vi "Inverter-DCread vi.vi"(0 "Numeric Control 6":dbl, 1 "Numeric Control 5":dbl, 2 "Numeric Control 4":dbl, 3 "Numeric Control 16":dbl, 4 "Numeric Control 15":dbl, 6 "Numeric Control 17":u32, 7 "Numeric Control 14":dbl, 8 "register values":u16[](array[numeric]), 9 "Numeric Control 13":dbl, 11 "Numeric Control 12":dbl) -> (10 "Numeric Control 3":dbl, 12 "Numeric Control 2":dbl, 13 "Numeric Control 7":dbl, 14 "Numeric Control":dbl, 15 "Numeric Control 10":dbl, 16 "Numeric Control 11":dbl, 17 "Numeric Control 9":dbl, 18 "Numeric Control 8":dbl)   [LabVIEW 2016]
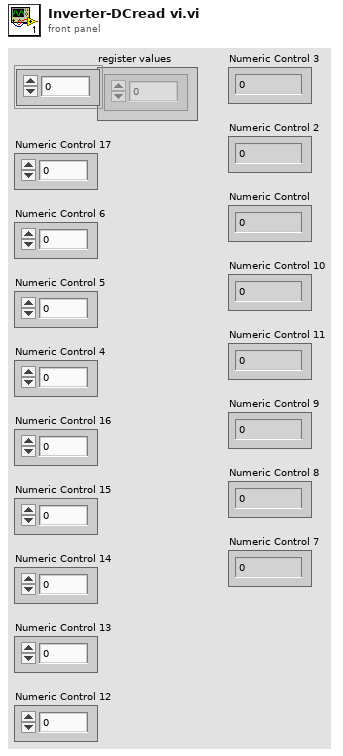
[diagram p1: front panel]
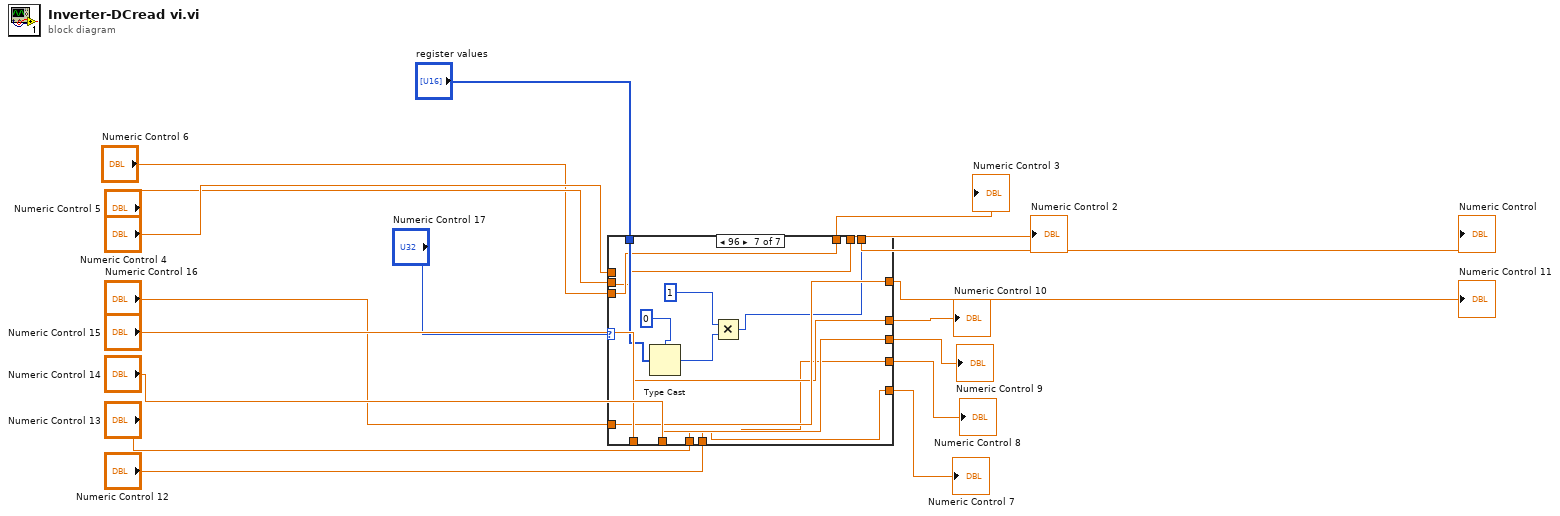
[diagram p0: block diagram]
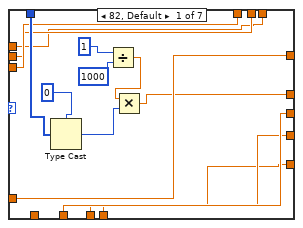
[diagram p2: hidden frame]
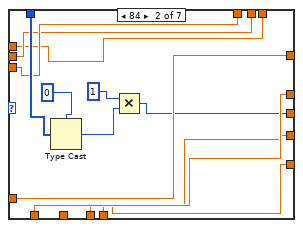
[diagram p3: hidden frame]
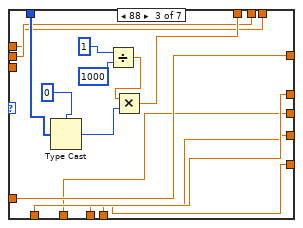
[diagram p4: hidden frame]
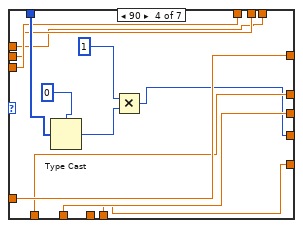
[diagram p5: hidden frame]
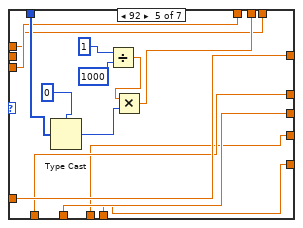
[diagram p6: hidden frame]
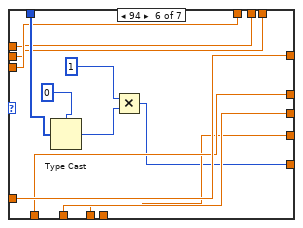
[diagram p7: hidden frame]
diagram:
  n1 = case shown="96" "Numeric Control 17" {
    tunnel: "register values" -> [w26 w41 w52 w67 w78 w93 w105]
    tunnel: [w29 w44 w55 w70 w81 w96 w108] -> w8
    tunnel: "Numeric Control 16" -> [w29 w44 w55 w70 w81 w96 w108]
    tunnel: [w19 w40 w51 w66 w77 w92 w104] -> w9
    tunnel: "Numeric Control 15" -> [_ w40 w51 w66 w77 w92 w104]
    tunnel: [w25 w39 w48 w65 w76 w91 w103] -> w10
    tunnel: "Numeric Control 14" -> [w25 _ w48 w65 w76 w91 w103]
    tunnel: [w24 w38 w50 w64 w73 w90 w102] -> w11
    tunnel: "Numeric Control 13" -> [w24 w38 w50 _ w73 w90 w102]
    tunnel: [w23 w37 w49 w63 w75 w89 w98] -> w12
    tunnel: "Numeric Control 12" -> [w23 w37 w49 w63 w75 _ w98]
    tunnel: [w22 w36 w47 w62 w74 w87 w100] -> w16
    tunnel: "Numeric Control 6" -> [w22 w36 _ w62 w74 w87 w100]
    tunnel: [w21 w35 w46 w61 w72 w86 w99] -> w17
    tunnel: "Numeric Control 5" -> [w21 w35 w46 w61 _ w86 w99]
    tunnel: [w20 w34 w45 w60 w71 w85 w97] -> w18
    tunnel: "Numeric Control 4" -> [w20 w34 w45 w60 w71 w85 _]
    frame 82, Default {
      n2 = Type Cast(type=0, x=w26) -> (*(type *) &x=w28:i32)
      n3 = Divide(x=u32 1, y=u32 1000) -> (x/y=w30:dbl)
      n4 = Multiply(x=w30, y=w28) -> (x*y=w19:dbl)
    }
    frame 84 {
      n5 = Type Cast(type=0, x=w41) -> (*(type *) &x=w43:i32)
      n6 = Multiply(x=u32 1, y=w43) -> (x*y=w39:u32)
    }
    frame 88 {
      n7 = Type Cast(type=u32 0, x=w52) -> (*(type *) &x=w54:u32)
      n8 = Divide(x=u32 1, y=u32 1000) -> (x/y=w56:dbl)
      n9 = Multiply(x=w56, y=w54) -> (x*y=w47:dbl)
    }
    frame 90 {
      n10 = Type Cast(type=u32 0, x=w67) -> (*(type *) &x=w69:u32)
      n11 = Multiply(x=u32 1, y=w69) -> (x*y=w64:u32)
    }
    frame 92 {
      n12 = Type Cast(type=u32 0, x=w78) -> (*(type *) &x=w80:u32)
      n13 = Divide(x=u32 1, y=u32 1000) -> (x/y=w82:dbl)
      n14 = Multiply(x=w82, y=w80) -> (x*y=w72:dbl)
    }
    frame 94 {
      n15 = Type Cast(type=u32 0, x=w93) -> (*(type *) &x=w95:u32)
      n16 = Multiply(x=1, y=w95) -> (x*y=w89:u32)
    }
    frame 96 {
      n17 = Type Cast(type=u16 0, x=w105) -> (*(type *) &x=w107:u16)
      n18 = Multiply(x=1, y=w107) -> (x*y=w97:i32)
    }
  }
  "Numeric Control" <- w18
  "Numeric Control 2" <- w17
  "Numeric Control 3" <- w16
  "Numeric Control 7" <- w12
  "Numeric Control 8" <- w11
  "Numeric Control 9" <- w10
  "Numeric Control 10" <- w9
  "Numeric Control 11" <- w8
